vi "Coerce fsync.vi"(8 "error in (no error)":errorcluster, 11 "session in":refnum<class "Session.lvclass">) -> (0 "error out":errorcluster, 3 "session out":refnum<class "Session.lvclass">)   [LabVIEW 2020, in "NI_SFTP.lvlib"]
uses:
  <vilib>/net/SFTP/NI_SFTP.lvlib
  <vilib>/net/SFTP/Session/Session.lvclass
  <vilib>/net/SFTP/Session/Session.lvclass/Session.ctl
  <vilib>/net/SFTP/Session/Read fsync.vi
  <vilib>/net/SFTP/Session/Write fsync.vi
  <vilib>/Utility/error.llb/Error Cluster From Error Code.vi
  <vilib>/ErrorRing/Error Ring.xnode
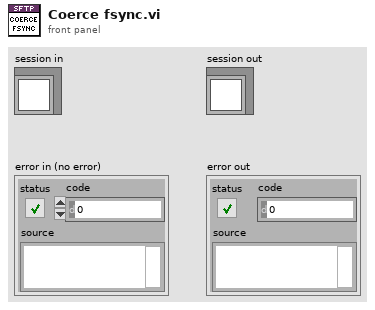
[diagram p1: front panel]
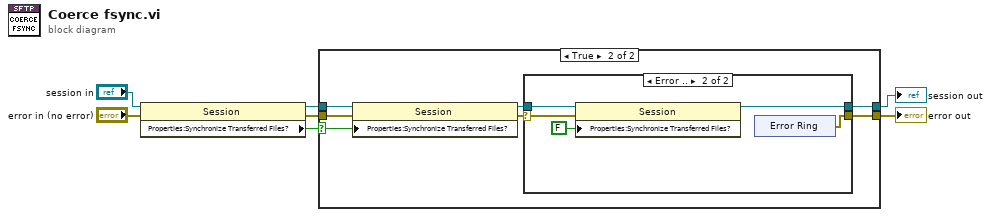
[diagram p0: block diagram]
diagram:
  n1 = property on="Property Node" class="Session"(reference="session in", error in="error in (no error)") -> (reference out=w4:refnum<class "Session.lvclass">, error out=w3:errorcluster, "Properties:Synchronize Transferred Files?"=w2:bool)
  n2 = case shown="True" w2 {
    selector: w2 -> [_ w16]
    tunnel: w3 -> [w8 w15]
    tunnel: w4 -> [w9 w14]
    tunnel: [w9 w11] -> w5
    tunnel: [w8 w10] -> w7
    frame False {
    }
    frame True {
      n3 = property on="Property Node" class="Session"(reference=w14, error in=w15, "Properties:Synchronize Transferred Files?"=w16) -> (reference out=w12:refnum<class "Session.lvclass">, error out=w13:errorcluster)
      n4 = case shown="Error .." w13 {
        selector: w13 -> [w17 w23]
        tunnel: w12 -> [w18 w22]
        tunnel: [w18 w20] -> w11
        tunnel: [w17 w19] -> w10
        frame No Error {
        }
        frame Error {
          n5 = property on="Property Node" class="Session"(reference=w22, error in=w23, "Properties:Synchronize Transferred Files?"=FALSE ("Synchronize Transferred Files?")) -> (reference out=w20:refnum<class "Session.lvclass">)  [unwired: 1 out]
          n6 = xnode ("Error Ring")() -> ("error out"=w19:errorcluster)
        }
      }
    }
  }
  "error out" <- w7
  "session out" <- w5
